vi "Interface_Asset_Get Parameter Control Refs.vi"(8 "error in (no error)":errorcluster, 11 "Load in":refnum<class "Load.lvclass">) -> (0 "error out":errorcluster, 2 "Controls[]":refnum<vi>[](array[refnum]), 3 "Load out":refnum<class "Load.lvclass">)   [LabVIEW 2015, in "Load.lvclass"]
uses:
  Load.lvclass
  Load_Status.ctl
  Load.lvclass/Load.ctl
panel:
  out "Status":T1
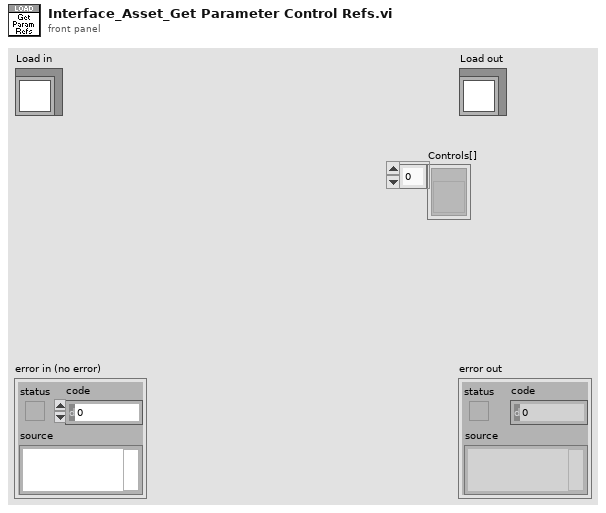
[diagram p1: front panel]
types:
  T1 = typedef "Load.lvclass/Load_Status.ctl" = cluster{"kW":dbl}
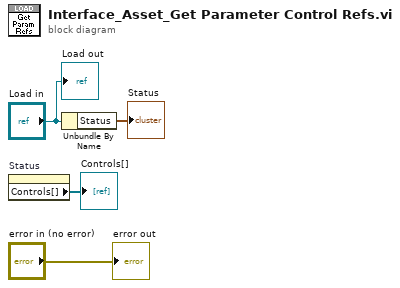
[diagram p0: block diagram]
diagram:
  n1 = property on="Status" class="Clust (strict)"() -> ("Controls[]"=→"Controls[]":refnum<vi>[])  [unwired: 2 in, 2 out]
  n2 = Unbundle By Name("Load in") -> ("Status"=→"Status":T1)
  "error out" <- "error in (no error)"
  "Load out" <- "Load in"
